vi "Managed Compressor.vi"(8 "Compressor Hysterisis":i16, 9 "Voltage threshold":dbl, 10 "Outside wait time (ms)":i16, 11 "Enum":enum16{"Start", "Run", "End"}(ring)) -> ()   [LabVIEW 2014]
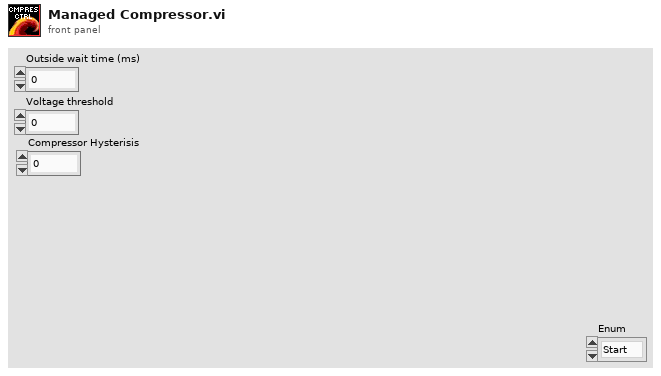
[diagram p1: front panel]
types:
  T1 = typedef "WPI_CompressorDevRef.ctl" = cluster{"DevStatus":errorcluster, "Pneumatics Control Module":u8}
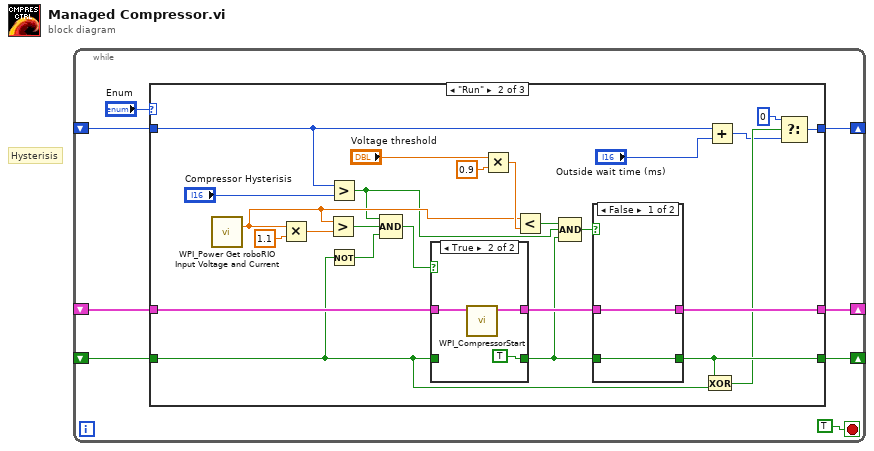
[diagram p0: block diagram]
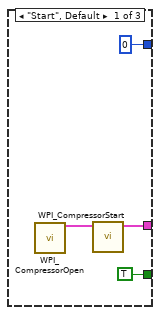
[diagram p2: hidden frame]
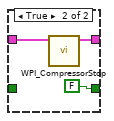
[diagram p4: hidden frame]
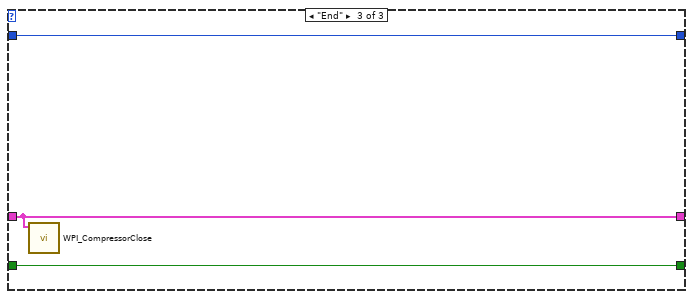
[diagram p5: hidden frame]
diagram:
  # "Hysterisis"
  n1 = while {
    shift-right: [w6] -> _
    shift-left: _ -> [w3]
    shift-right: [w5] -> _
    shift-left: _ -> [w4]
    shift-right: [w2] -> _
    shift-left: _ -> [w1]
    stop <- TRUE stop-if-true
    n2 = case shown="\"Run\"" "Enum" {
      tunnel: [w11 w34 w50] -> w6
      tunnel: [i16 0 w21 w49] -> w5
      tunnel: w4 -> [_ w18 w49]
      tunnel: w3 -> [_ w36 w50]
      tunnel: [TRUE w25 w48] -> w2
      tunnel: w1 -> [_ w24 w48]
      frame "Start", Default {
        n3 = call <vilib>:"WPI_CompressorOpen.vi"() -> ("CompressorDevRef"=w12:T1)  [unwired: 14 in, 1 out]
        n4 = call <vilib>:"WPI_CompressorStart.vi"("CompressorDevRef"=w12) -> ("CompressorDevRef"=w11:T1)  [unwired: 9 in, 1 out]
      }
      frame "Run" {
        n5 = call <vilib>:"WPI_Power Get roboRIO Input Voltage and Current.vi"() -> ("roboRIO input voltage (V)"=w19:dbl)  [unwired: 13 in, 2 out]
        n6 = Multiply(x=w19, y=1.1) -> (x*y=w31:dbl)
        n7 = Greater?(x=w19, y=w31) -> (0:w33:bool)
        n8 = Greater?(x=w18, y="Compressor Hysterisis") -> (0:w14:bool)
        n9 = Not(x=w24) -> (.not. x?=w16:bool)
        n10 = Compound Arithmetic op=AND(w14, w33, w16) -> (w26:bool)
        n11 = case shown="True" w26 {
          tunnel: w36 -> [w39 w42]
          tunnel: [w39 w41] -> w35
          tunnel: [w38 TRUE] -> w13
          tunnel: w24 -> [w38 _]
          frame False {
          }
          frame True {
            n12 = call <vilib>:"WPI_CompressorStart.vi"("CompressorDevRef"=w42) -> ("CompressorDevRef"=w41:T1)  [unwired: 9 in, 1 out]
          }
        }
        n13 = Multiply(x="Voltage threshold", y=0.9) -> (x*y=w28:dbl)
        n14 = Less?(x=w19, y=w28) -> (x < y?=w15:bool)
        n15 = Compound Arithmetic op=AND(w15, w14, w13) -> (w27:bool)
        n16 = case shown="False" w27 {
          tunnel: w35 -> [w44 w47]
          tunnel: [w44 w46] -> w34
          tunnel: w13 -> [w43 _]
          tunnel: [w43 FALSE] -> w25
          frame False {
          }
          frame True {
            n17 = call <vilib>:"WPI_CompressorStop.vi"("CompressorDevRef"=w47) -> ("CompressorDevRef"=w46:T1)  [unwired: 9 in, 1 out]
          }
        }
        n18 = Exclusive Or(1:w24, 2:w25) -> (0:w23:bool)
        n19 = Add(x=w18, y="Outside wait time (ms)") -> (x+y=w22:i16)
        n20 = Select(t=i16 0, s=w23, f=w22) -> (s? t:f=w21:i16)
      }
      frame "End" {
        n21 = call <vilib>:"WPI_CompressorClose.vi"("CompressorDevRef"=w50) -> ()  [unwired: 10 in, 1 out]
      }
    }
  }
